vi "Test_AutoStateMachine.vi"() -> ()   [LabVIEW 2017]
panel:
  out "String":string
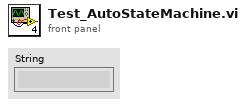
[diagram p1: front panel]
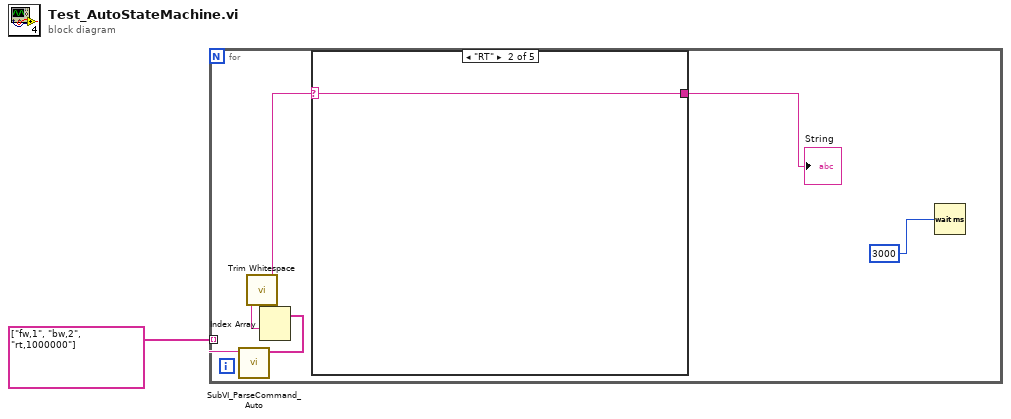
[diagram p0: block diagram]
diagram:
  n1 = for {
    tunnel: string[] ["fw,1", "bw,2", "rt,1000000"] ("String Array") -> [w7] mode=indexing
    n2 = call "SubVI_ParseCommand_Auto.vi"("String"=w7) -> ("array"=w6:string[])  [unwired: 10 in]
    n3 = Index Array(array=w6) -> (element #1=w5:string)  [unwired: 2 in, 1 out]
    n4 = call <vilib>:"Trim Whitespace.vi"("string"=w5) -> ("trimmed string"=w4:string)  [unwired: 1 in]
    n5 = case shown="\"RT\"" w4 {
      selector: w4 -> [w8 w9 w10 w11 w12]
      tunnel: [w8 w9 w10 w11 w12] -> w3
      frame "LT" {
      }
      frame "RT" {
      }
      frame "FW" {
      }
      frame "de", Default {
      }
      frame "BW" {
      }
    }
    "String" <- w3
    n6 = Wait (ms)(milliseconds to wait=u32 3000 ("millisecond timer value")) -> ()  [unwired: 1 out]
  }
